vi "Minima_to_Minima (SubVI).vi"(11 "Y":dbl[](array[numeric])) -> (0 "length":dbl, 1 "index":i32, 3 "Array":dbl[](array[numeric]))   [LabVIEW 2017]
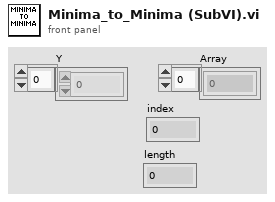
[diagram p1: front panel]
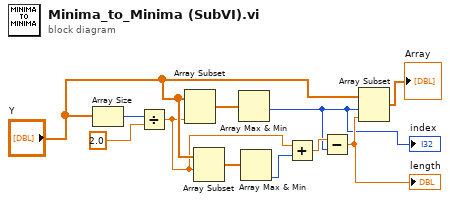
[diagram p0: block diagram]
diagram:
  n1 = Array Size(array="Y") -> (size(s)=w2:i32)
  n2 = Divide(x=w2, y=2.0 ("Min Value")) -> (x/y=w7:dbl)
  n3 = Array Subset(array="Y", length=w7) -> (w3:dbl[])  [unwired: 1 in]
  n4 = Array Subset(array="Y", index=w7) -> (w5:dbl[])  [unwired: 1 in]
  n5 = Array Max & Min(array=w3) -> (min index (indices)=w1:i32)  [unwired: 3 out]
  "index" <- w1
  n6 = Array Max & Min(array=w5) -> (min index (indices)=w6:i32)  [unwired: 3 out]
  n7 = Add(x=w7, y=w6) -> (x+y=w8:dbl)
  n8 = Subtract(x=w8, y=w1) -> (x-y=w9:dbl)
  "length" <- w9
  n9 = Array Subset(array="Y", index=w1, length=w9) -> (→"Array":dbl[])
